vi "Main.vi"(8 "error in (no error)":errorcluster, 11 "ImageStackBase in":refnum<class "ImageStack.lvclass">) -> (0 "error out":errorcluster, 3 "component":refnum<class "ImageStack.lvclass">)   [LabVIEW 2012, in "ImageStack.lvclass"]
doc: "Main VI of the component."
uses:
  ImageStack.lvclass
  <vilib>/Distrio/Murmex/Murmex/command_enum.ctl
  ImageStack.lvclass/ImageStack.ctl
  <vilib>/Distrio/Murmex/InitialiseMessage/InitialiseMessage.lvclass
  <vilib>/Distrio/Murmex/Murmex/data_compression_enum.ctl
  <vilib>/Distrio/Murmex/TerminateMessage/TerminateMessage.lvclass
  <vilib>/Distrio/Murmex/ConfigureMessage/ConfigureMessage.lvclass
  <vilib>/Distrio/Murmex/Murmex/update_cluster.ctl
  <vilib>/Distrio/Murmex/StartMessage/StartMessage.lvclass
  <vilib>/Distrio/Murmex/StopMessage/StopMessage.lvclass
  <vilib>/Distrio/Murmex/Murmex/Set configure at initialise.vi
  <vilib>/Distrio/Murmex/Murmex/Set log reference.vi
  <vilib>/Distrio/Murmex/Murmex/Set VI reference.vi
  <vilib>/Distrio/Murmex/Murmex/Set relay start stop to observers.vi
  <vilib>/Distrio/Murmex/Murmex/Set data compression.vi
  <vilib>/Distrio/Murmex/Murmex/Murmex.lvclass
  <vilib>/Distrio/Murmex/Message/Message.lvclass
panel:
  in  "button:config":bool
  in  "Tab Control":enum32{"User", "Debug", "About"}(tab)
  in  "button::direction":bool
  in  "File name":string
  out "Translation speed":dbl[unit]
  in  "button:start":bool
  in  "No. of frames":u16=100
  out "Frame rate":dbl[unit]
  in  "Subfolder levels":string[](array[string])
  in  "Step size":dbl[unit]
  out "log":string
  in  "ID":string
  in  "button:send command":bool
  in  "Generic command":string
  in  "command":T1
  in  "button:quit":bool
  in  "terminate?":bool=TRUE
  # "ImageStack\n\nImplemented by:\nLudovico Silvestri\nUniversity of Florence, Italy"
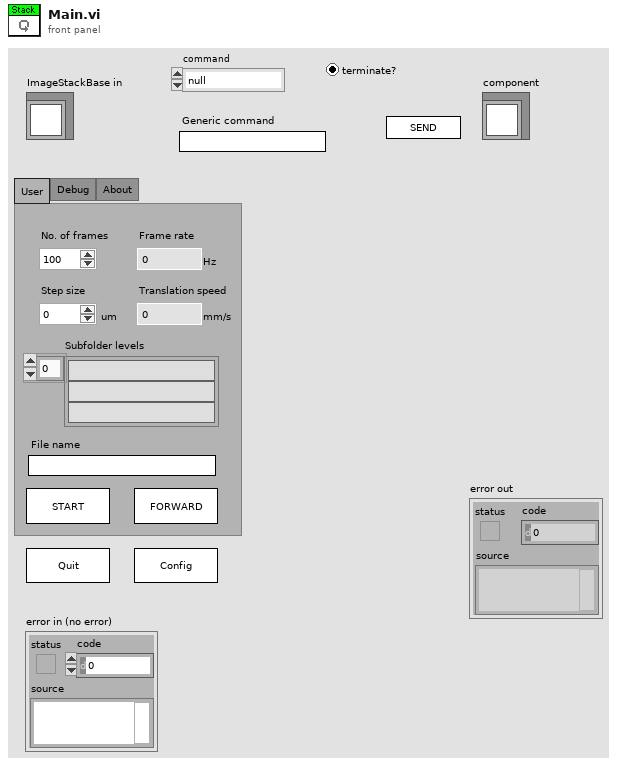
[diagram p1: front panel]
types:
  T1 = typedef "Murmex.lvlib/Murmex.lvclass/command_enum.ctl" = enum16{"null", "initialise", "reset", "terminate", "acknowledge", "update", "inspect", "inform", "proceed", "start", "stop", "fetch", "configure", "generic"}
  T2 = typedef "Murmex.lvlib/Murmex.lvclass/data_compression_enum.ctl" = enum16{"base64", "zip+base64", "byte to string"}
  T3 = typedef "Murmex.lvlib/Murmex.lvclass/update_cluster.ctl" = cluster{"target ID":string, "key chains":string[], "values":variant[]}
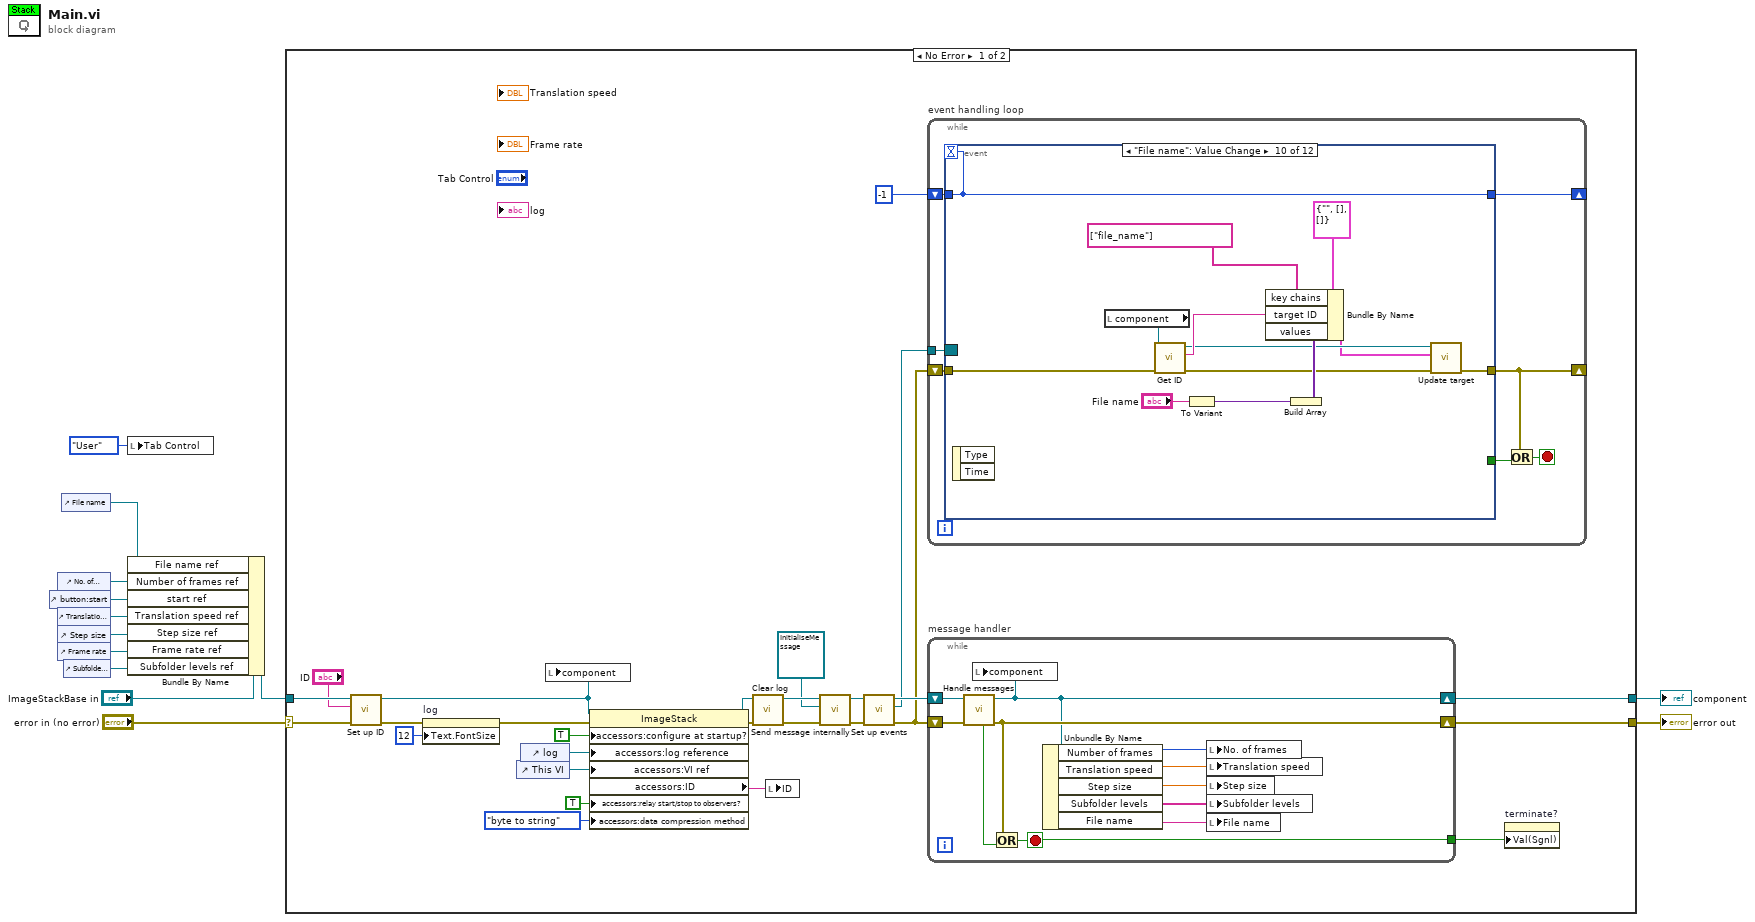
[diagram p0: block diagram]
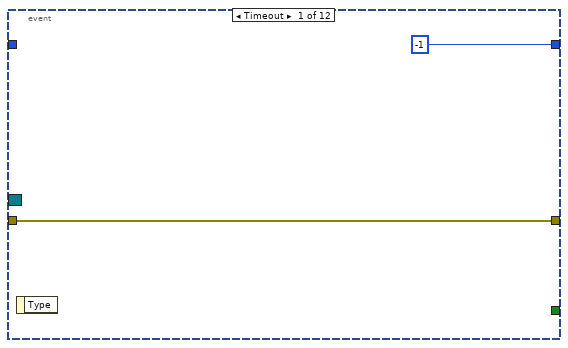
[diagram p2: hidden frame]
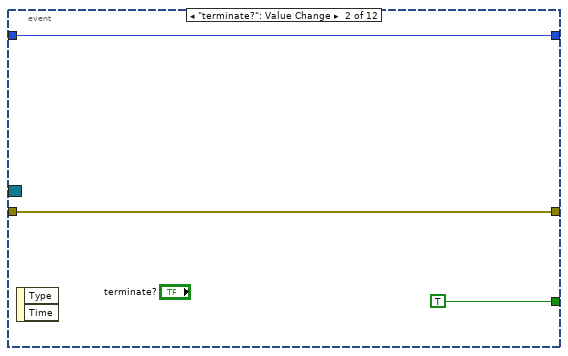
[diagram p3: hidden frame]
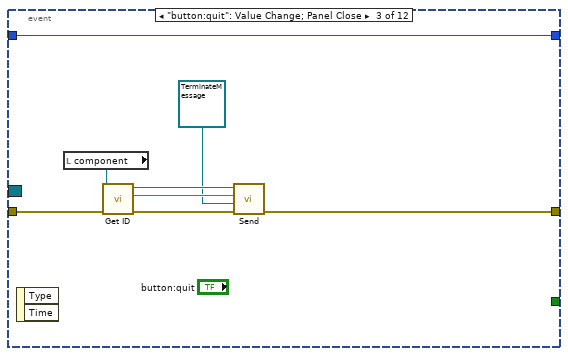
[diagram p4: hidden frame]
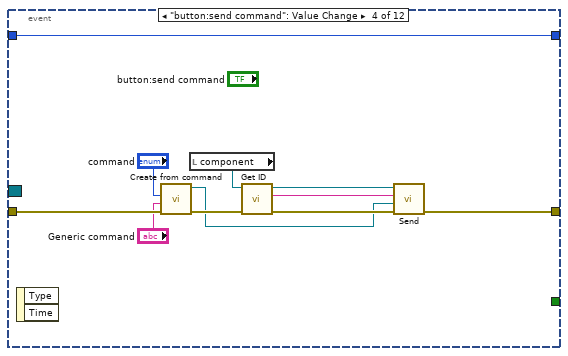
[diagram p5: hidden frame]
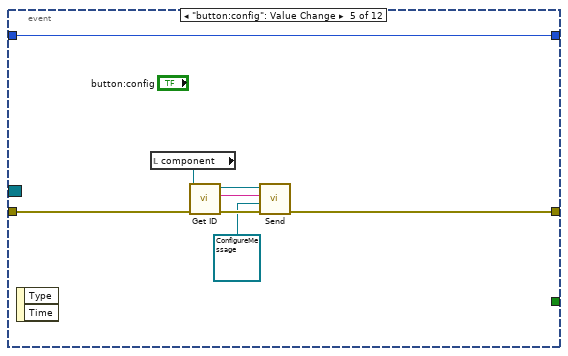
[diagram p6: hidden frame]
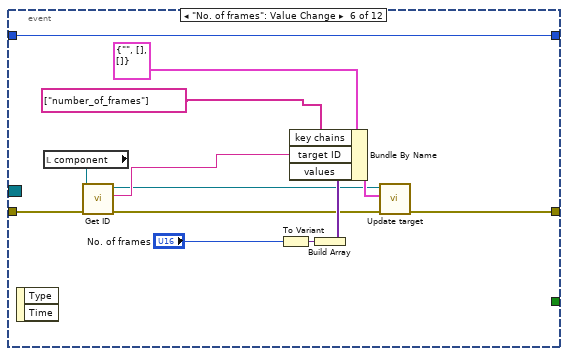
[diagram p7: hidden frame]
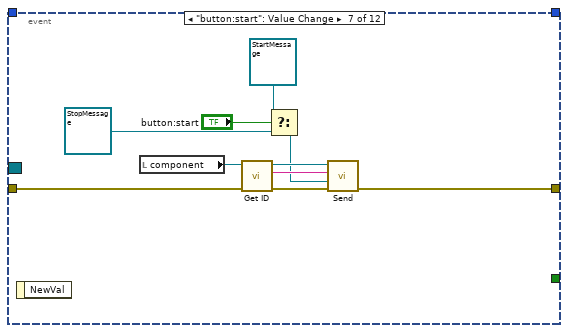
[diagram p8: hidden frame]
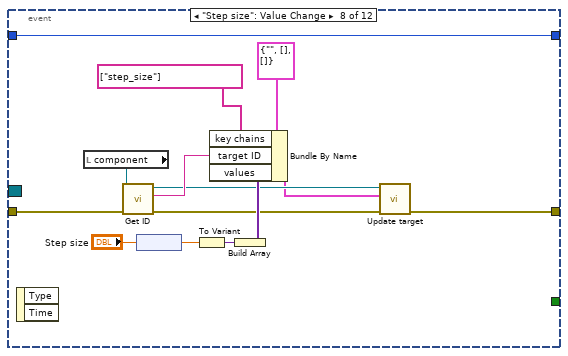
[diagram p9: hidden frame]
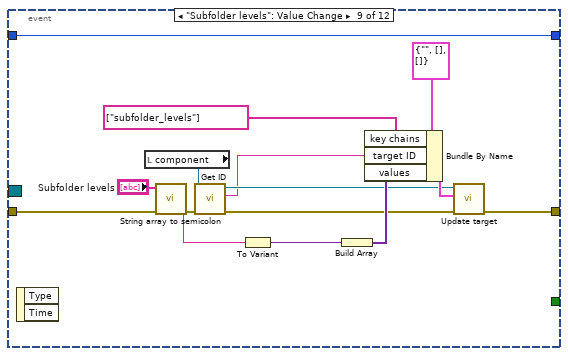
[diagram p10: hidden frame]
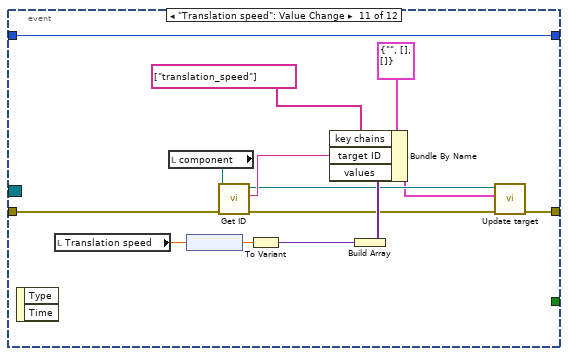
[diagram p11: hidden frame]
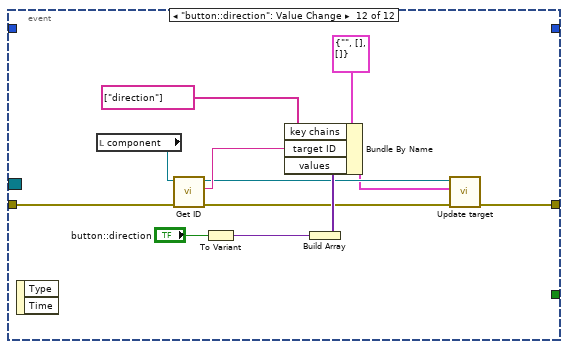
[diagram p12: hidden frame]
diagram:
  n1 = control-ref of="button:start"() -> (w4:refnum<vi>)
  n2 = control-ref of="No. of frames"() -> (w3:refnum<vi>)
  n3 = control-ref of="Translation speed"() -> (w5:refnum<vi>)
  n4 = control-ref of="Step size"() -> (w6:refnum<vi>)
  n5 = control-ref of="Frame rate"() -> (w7:refnum<vi>)
  n6 = control-ref of="File name"() -> (w1:refnum<vi>)
  n7 = control-ref of="Subfolder levels"() -> (w8:refnum<vi>)
  n8 = local write "Tab Control"(enum32{"User", "Debug", "About"}."User" ("Tab Control")) -> ()
  n9 = Bundle By Name(cluster="ImageStackBase in", "File name ref"=w1, "Number of frames ref"=w3, "start ref"=w4, "Translation speed ref"=w5, "Step size ref"=w6, "Frame rate ref"=w7, "Subfolder levels ref"=w8) -> (w9:refnum<class "ImageStack.lvclass">)
  n10 = case shown="No Error" "error in (no error)" {
    selector: "error in (no error)" -> [w32 w182]
    tunnel: w9 -> [w31 w183]
    tunnel: [w24 w183] -> w11
    tunnel: [w23 w182] -> w10
    frame No Error {
      n11 = call <vilib>:"Set up ID.vi"("error in (no error)"=w32, "component ID"="ID", "MurmexBase in"=w31) -> ("error out"=w18:errorcluster, "MurmexBase out"=w28:refnum<class "ImageStack.lvclass">)  [unwired: 6 in, 1 out]
      n12 = property on="log" class="Str"(error in=w18, "Text.FontSize"=u32 12 ("Text.Font:Size")) -> (error out=w17:errorcluster)  [unwired: 1 in, 1 out]
      n13 = control-ref of="This VI"() -> (w38:refnum<vi>)
      n14 = control-ref of="log"() -> (w39:refnum<vi>)
      n15 = local write "component"(w28) -> ()
      n16 = property class="ImageStack"(reference=w28, error in=w17, "accessors:configure at startup?"=TRUE ("configure at startup?"), "accessors:log reference"=w39, "accessors:VI ref"=w38, "accessors:relay start/stop to observers?"=TRUE ("relay start/stop to observers?"), "accessors:data compression method"=data_compression_enum."byte to string" ("data compression method")) -> (reference out=w37:refnum<class "ImageStack.lvclass">, error out=w36:errorcluster, "accessors:ID"=w29:string)
      n17 = call <vilib>:"Clear log.vi"("error in (no error)"=w36, "MurmexBase in"=w37) -> ("error out"=w35:errorcluster, "MurmexBase out"=w34:refnum<class "ImageStack.lvclass">)  [unwired: 8 in]
      n18 = local write "ID"(w29) -> ()
      n19 = call <vilib>:"Send message internally.vi"("error in (no error)"=w35, "Message"=refnum<class "InitialiseMessage.lvclass"> refnum ("Murmex.lvlib:InitialiseMessage"), "Murmex in"=w34) -> ("error out"=w27:errorcluster, "Murmex out"=w26:refnum<class "ImageStack.lvclass">)  [unwired: 7 in]
      n20 = call <vilib>:"Set up events.vi"("error in (no error)"=w27, "MurmexBase in"=w26) -> ("error out"=w21:errorcluster, "Event Registration Refnum"=w20:refnum<event-registration>, "MurmexBase out"=w25:refnum<class "ImageStack.lvclass">)  [unwired: 7 in]
      n21 = while "event handling loop" {
        shift-right: [w46] -> _
        shift-left: -1 -> [w47]
        shift-right: [w42] -> _
        shift-left: w21 -> [w45]
        tunnel: w20 -> [w44]
        stop <- w43 stop-if-true
        n22 = event shown="[9] \"File name\": Value Change" {
          selector: w44 -> [_ _ _ _ _ _ _ _ _ _ _ _]
          dyn-events: _ -> [_ _ _ _ _ _ _ _ _ _ _ _]
          timeout: w47 -> [_ _ _ _ _ _ _ _ _ _ _ _]
          tunnel: w47 -> [_ w50 w53 w61 w72 w88 _ w104 w126 w134 w148 _]
          tunnel: [-1 w50 w53 w61 w72 w88 _ w104 w126 w134 w148 _] -> w46
          tunnel: [w48 w52 w56 w66 w77 w89 w97 w108 w127 w137 w151 w160] -> w42
          tunnel: w45 -> [w48 w52 w60 w71 w79 w91 w98 w114 w125 w133 w147 w162]
          tunnel: [_ TRUE _ _ _ _ _ _ _ _ _ _] -> w41
          event Timeout {
            n23 = event-data() -> ()  [unwired: 1 in, 1 out]
          }
          event "terminate?": Value Change {
            n24 = event-data() -> ()  [unwired: 1 in, 2 out]
          }
          event "button:quit": Value Change; Panel Close {
            n25 = event-data() -> ()  [unwired: 1 in, 2 out]
            n26 = local read "component"() -> (w59:refnum<class "ImageStack.lvclass">)
            n27 = call <vilib>:"Get ID.vi"("error in (no error)"=w60, "Murmex in"=w59) -> ("error out"=w57:errorcluster, "component id"=w55:string, "Murmex out"=w58:refnum<class "ImageStack.lvclass">)  [unwired: 7 in]
            n28 = call <vilib>:"Send.vi"("error in (no error)"=w57, "Message"=refnum<class "TerminateMessage.lvclass"> refnum ("Murmex.lvlib:TerminateMessage"), "recipient"=w55, "Murmex in"=w58) -> ("error out"=w56:errorcluster)  [unwired: 6 in, 1 out]
          }
          event "button:send command": Value Change {
            n29 = event-data() -> ()  [unwired: 1 in, 2 out]
            n30 = call <vilib>:"Create from command.vi"("error in (no error)"=w71, "generic command"="Generic command", "command"="command") -> ("error out"=w68:errorcluster, "Message out"=w65:refnum<class "Message.lvclass">)  [unwired: 7 in]
            n31 = local read "component"() -> (w64:refnum<class "ImageStack.lvclass">)
            n32 = call <vilib>:"Get ID.vi"("error in (no error)"=w68, "Murmex in"=w64) -> ("error out"=w67:errorcluster, "component id"=w62:string, "Murmex out"=w63:refnum<class "ImageStack.lvclass">)  [unwired: 7 in]
            n33 = call <vilib>:"Send.vi"("error in (no error)"=w67, "Message"=w65, "recipient"=w62, "Murmex in"=w63) -> ("error out"=w66:errorcluster)  [unwired: 6 in, 1 out]
          }
          event "button:config": Value Change {
            n34 = event-data() -> ()  [unwired: 1 in, 2 out]
            n35 = local read "component"() -> (w73:refnum<class "ImageStack.lvclass">)
            n36 = call <vilib>:"Get ID.vi"("error in (no error)"=w79, "Murmex in"=w73) -> ("error out"=w78:errorcluster, "component id"=w75:string, "Murmex out"=w76:refnum<class "ImageStack.lvclass">)  [unwired: 7 in]
            n37 = call <vilib>:"Send.vi"("error in (no error)"=w78, "Message"=refnum<class "ConfigureMessage.lvclass"> refnum ("Murmex.lvlib:ConfigureMessage"), "recipient"=w75, "Murmex in"=w76) -> ("error out"=w77:errorcluster)  [unwired: 6 in, 1 out]
          }
          event "No. of frames": Value Change {
            n38 = event-data() -> ()  [unwired: 1 in, 2 out]
            n39 = local read "component"() -> (w90:refnum<class "ImageStack.lvclass">)
            n40 = call <vilib>:"Get ID.vi"("error in (no error)"=w91, "Murmex in"=w90) -> ("error out"=w80:errorcluster, "component id"=w82:string, "Murmex out"=w81:refnum<class "ImageStack.lvclass">)  [unwired: 7 in]
            n41 = To Variant(anything="No. of frames") -> (Variant=w85:variant)
            n42 = Build Array(w85) -> (w84:variant[])
            n43 = Bundle By Name(cluster=T3 {"target ID"="", "key chains"=[], "values"=[]} ("update cluster"), "key chains"=string[] ["number_of_frames"], "target ID"=w82, "values"=w84) -> (w83:T3)
            n44 = call <vilib>:"Update target.vi"("error in (no error)"=w80, "update cluster"=w83, "MurmexBase in"=w81) -> ("error out"=w89:errorcluster)  [unwired: 7 in, 1 out]
          }
          event "button:start": Value Change {
            n45 = event-data() -> ()  [unwired: 1 in, 1 out]
            n46 = local read "component"() -> (w99:refnum<class "ImageStack.lvclass">)
            n47 = call <vilib>:"Get ID.vi"("error in (no error)"=w98, "Murmex in"=w99) -> ("error out"=w102:errorcluster, "component id"=w100:string, "Murmex out"=w101:refnum<class "ImageStack.lvclass">)  [unwired: 7 in]
            n48 = Select(t=refnum<class "StartMessage.lvclass"> refnum ("Message in"), s="button:start", f=refnum<class "StopMessage.lvclass"> refnum ("Distrio Murmex 1.0:StopMessage")) -> (s? t:f=w94:refnum<class "Message.lvclass">)
            n49 = call <vilib>:"Send.vi"("error in (no error)"=w102, "Message"=w94, "recipient"=w100, "Murmex in"=w101) -> ("error out"=w97:errorcluster)  [unwired: 6 in, 1 out]
          }
          event "Step size": Value Change {
            n50 = event-data() -> ()  [unwired: 1 in, 2 out]
            n51 = local read "component"() -> (w110:refnum<class "ImageStack.lvclass">)
            n52 = call <vilib>:"Get ID.vi"("error in (no error)"=w114, "Murmex in"=w110) -> ("error out"=w109:errorcluster, "component id"=w113:string, "Murmex out"=w107:refnum<class "ImageStack.lvclass">)  [unwired: 7 in]
            n53 = node("Step size") -> (w103:dbl)
            n54 = To Variant(anything=w103) -> (Variant=w112:variant)
            n55 = Build Array(w112) -> (w111:variant[])
            n56 = Bundle By Name(cluster=T3 {"target ID"="", "key chains"=[], "values"=[]} ("update cluster"), "key chains"=string[] ["step_size"], "target ID"=w113, "values"=w111) -> (w106:T3)
            n57 = call <vilib>:"Update target.vi"("error in (no error)"=w109, "update cluster"=w106, "MurmexBase in"=w107) -> ("error out"=w108:errorcluster)  [unwired: 7 in, 1 out]
          }
          event "Subfolder levels": Value Change {
            n58 = event-data() -> ()  [unwired: 1 in, 2 out]
            n59 = local read "component"() -> (w128:refnum<class "ImageStack.lvclass">)
            n60 = call "String array to semicolon.vi"("error in"=w125, "String array"="Subfolder levels") -> ("error out"=w124:errorcluster, "Semicolon string"=w122:string)  [unwired: 8 in]
            n61 = call <vilib>:"Get ID.vi"("error in (no error)"=w124, "Murmex in"=w128) -> ("error out"=w118:errorcluster, "component id"=w117:string, "Murmex out"=w119:refnum<class "ImageStack.lvclass">)  [unwired: 7 in]
            n62 = To Variant(anything=w122) -> (Variant=w129:variant)
            n63 = Build Array(w129) -> (w121:variant[])
            n64 = Bundle By Name(cluster=T3 {"target ID"="", "key chains"=[], "values"=[]} ("update cluster"), "key chains"=string[] ["subfolder_levels"], "target ID"=w117, "values"=w121) -> (w120:T3)
            n65 = call <vilib>:"Update target.vi"("error in (no error)"=w118, "update cluster"=w120, "MurmexBase in"=w119) -> ("error out"=w127:errorcluster)  [unwired: 7 in, 1 out]
          }
          event "File name": Value Change {
            n66 = event-data() -> ()  [unwired: 1 in, 2 out]
            n67 = local read "component"() -> (w139:refnum<class "ImageStack.lvclass">)
            n68 = call <vilib>:"Get ID.vi"("error in (no error)"=w133, "Murmex in"=w139) -> ("error out"=w138:errorcluster, "component id"=w142:string, "Murmex out"=w136:refnum<class "ImageStack.lvclass">)  [unwired: 7 in]
            n69 = To Variant(anything="File name") -> (Variant=w141:variant)
            n70 = Build Array(w141) -> (w140:variant[])
            n71 = Bundle By Name(cluster=T3 {"target ID"="", "key chains"=[], "values"=[]} ("update cluster"), "key chains"=string[] ["file_name"], "target ID"=w142, "values"=w140) -> (w135:T3)
            n72 = call <vilib>:"Update target.vi"("error in (no error)"=w138, "update cluster"=w135, "MurmexBase in"=w136) -> ("error out"=w137:errorcluster)  [unwired: 7 in, 1 out]
          }
          event "Translation speed": Value Change {
            n73 = event-data() -> ()  [unwired: 1 in, 2 out]
            n74 = local read "Translation speed"() -> (w146:dbl[unit])
            n75 = local read "component"() -> (w153:refnum<class "ImageStack.lvclass">)
            n76 = node(w146) -> (w145:dbl)
            n77 = call <vilib>:"Get ID.vi"("error in (no error)"=w147, "Murmex in"=w153) -> ("error out"=w152:errorcluster, "component id"=w156:string, "Murmex out"=w150:refnum<class "ImageStack.lvclass">)  [unwired: 7 in]
            n78 = To Variant(anything=w145) -> (Variant=w155:variant)
            n79 = Build Array(w155) -> (w154:variant[])
            n80 = Bundle By Name(cluster=T3 {"target ID"="", "key chains"=[], "values"=[]} ("update cluster"), "key chains"=string[] ["translation_speed"], "target ID"=w156, "values"=w154) -> (w149:T3)
            n81 = call <vilib>:"Update target.vi"("error in (no error)"=w152, "update cluster"=w149, "MurmexBase in"=w150) -> ("error out"=w151:errorcluster)  [unwired: 7 in, 1 out]
          }
          event "button::direction": Value Change {
            n82 = event-data() -> ()  [unwired: 1 in, 2 out]
            n83 = local read "component"() -> (w161:refnum<class "ImageStack.lvclass">)
            n84 = call <vilib>:"Get ID.vi"("error in (no error)"=w162, "Murmex in"=w161) -> ("error out"=w166:errorcluster, "component id"=w169:string, "Murmex out"=w165:refnum<class "ImageStack.lvclass">)  [unwired: 7 in]
            n85 = To Variant(anything="button::direction") -> (Variant=w168:variant)
            n86 = Build Array(w168) -> (w167:variant[])
            n87 = Bundle By Name(cluster=T3 {"target ID"="", "key chains"=[], "values"=[]} ("update cluster"), "key chains"=string[] ["direction"], "target ID"=w169, "values"=w167) -> (w164:T3)
            n88 = call <vilib>:"Update target.vi"("error in (no error)"=w166, "update cluster"=w164, "MurmexBase in"=w165) -> ("error out"=w160:errorcluster)  [unwired: 7 in, 1 out]
          }
        }
        n89 = Or(x=w42, y=w41) -> (x .or. y?=w43:bool)
      }
      n90 = while "message handler" {
        shift-right: [w176] -> w24
        shift-left: w25 -> [w181]
        shift-right: [w179] -> w23
        shift-left: w21 -> [w180]
        tunnel: [w177] -> w19
        stop <- w177 stop-if-true
        n91 = call <vilib>:"Handle messages.vi"("error in (no error)"=w180, "Murmex in"=w181) -> ("error out"=w179:errorcluster, "Murmex out"=w176:refnum<class "ImageStack.lvclass">, "terminated?"=w178:bool)  [unwired: 7 in]
        n92 = local write "component"(w176) -> ()
        n93 = Or(x=w179, y=w178) -> (x .or. y?=w177:bool)
        n94 = Unbundle By Name(w176) -> ("Number of frames"=w174:u16, "Translation speed"=w175:dbl[unit], "Step size"=w173:dbl[unit], "Subfolder levels"=w172:string[], "File name"=w171:string)
        n95 = local write "No. of frames"(w174) -> ()
        n96 = local write "Translation speed"(w175) -> ()
        n97 = local write "Step size"(w173) -> ()
        n98 = local write "Subfolder levels"(w172) -> ()
        n99 = local write "File name"(w171) -> ()
      }
      n100 = property on="terminate?" class="Bool (strict)"("Val(Sgnl)"=w19) -> ()  [unwired: 2 in, 2 out]
    }
    frame Error {
    }
  }
  "error out" <- w10
  "component" <- w11
